vi "Process.vi"(11 "Actor":refnum<class "Alarm Handler Actor.lvclass">) -> ()   [LabVIEW 2015, in "Alarm Handler Actor.lvclass"]
uses:
  Alarm Handler Actor.lvclass
  Re-use Libraries/Utility/UI/System Button (without mouse hover).ctl
  Re-use Libraries/Minimal Actor Framework/Actors/Base Actor/Actor/Front Panel State.ctl
  Alarm Handler Actor.lvclass/Alarm Handler Actor.ctl
  Re-use Libraries/Utility/Utility.lvlib
  Re-use Libraries/Minimal Actor Framework/Actors/Base Actor/Actor/Actor.lvclass
  Re-use Libraries/Minimal Actor Framework/Messaging/Message/Message.lvclass
panel:
  out "Detail":string
  in  "Acknowledge":T1
  out "Number Of Errors":i32
  in  "Alarms":i32(listbox)=-1
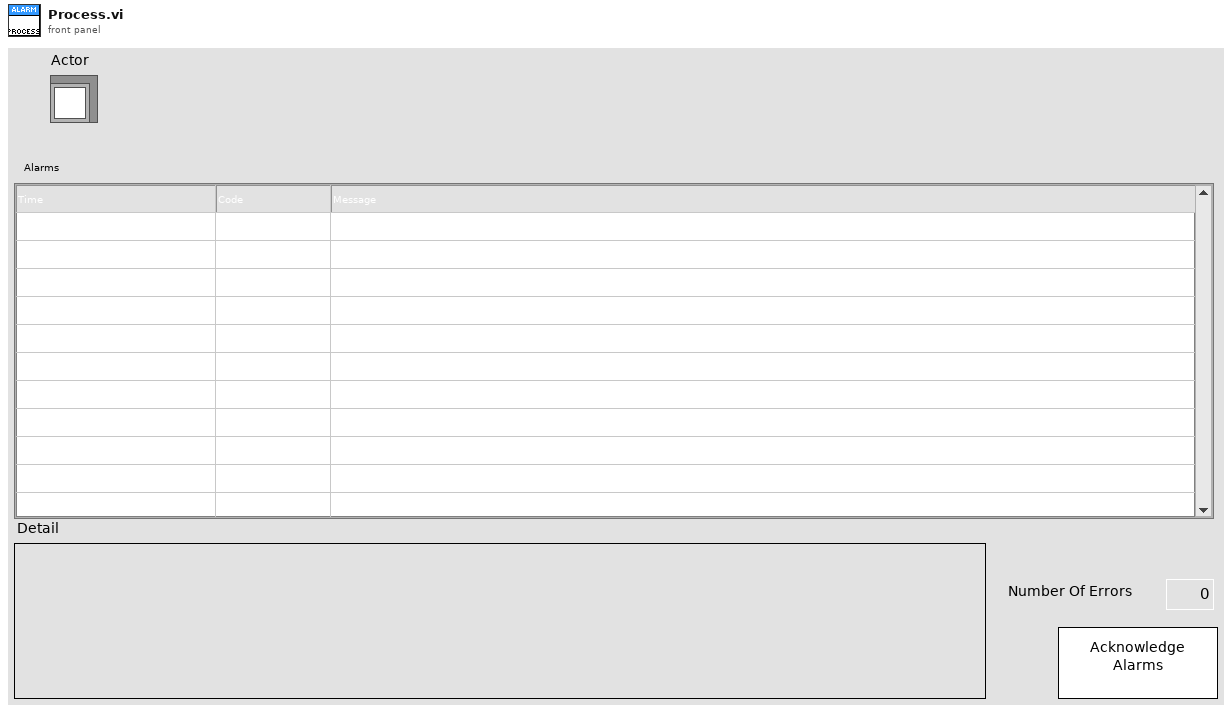
[diagram p1: front panel]
types:
  T1 = typedef "Utility.lvlib/System Button (without mouse hover).ctl" = bool
  T2 = typedef "Actor.lvclass/Front Panel State.ctl" = enum32{"Invalid", "Standard", "Closed", "Hidden", "Minimized", "Maximized"}
  T3 = typedef "LVPoint32TypeDef.ctl" = cluster{"Horizontal":i32, "Vertical":i32}
  T4 = typedef "LVRowAndColumnTypeDef.ctl" = cluster{"Row":i32, "Column":i32}
  T5 = typedef "Alarm Handler Actor.lvclass/Active Alarm.ctl" = cluster{"Alarm Detail":T6, "Count":i32, "First Error":timestamp, "Last Error":timestamp, "LabVIEW Error":bool}
  T6 = typedef "Alarm Handler Actor.lvclass/Alarm Details.ctl" = cluster{"Code":i32, "Loop":i32, "Description":string, "Severity":i32, "Clear on Ack?":bool, "Log All Events?":bool}
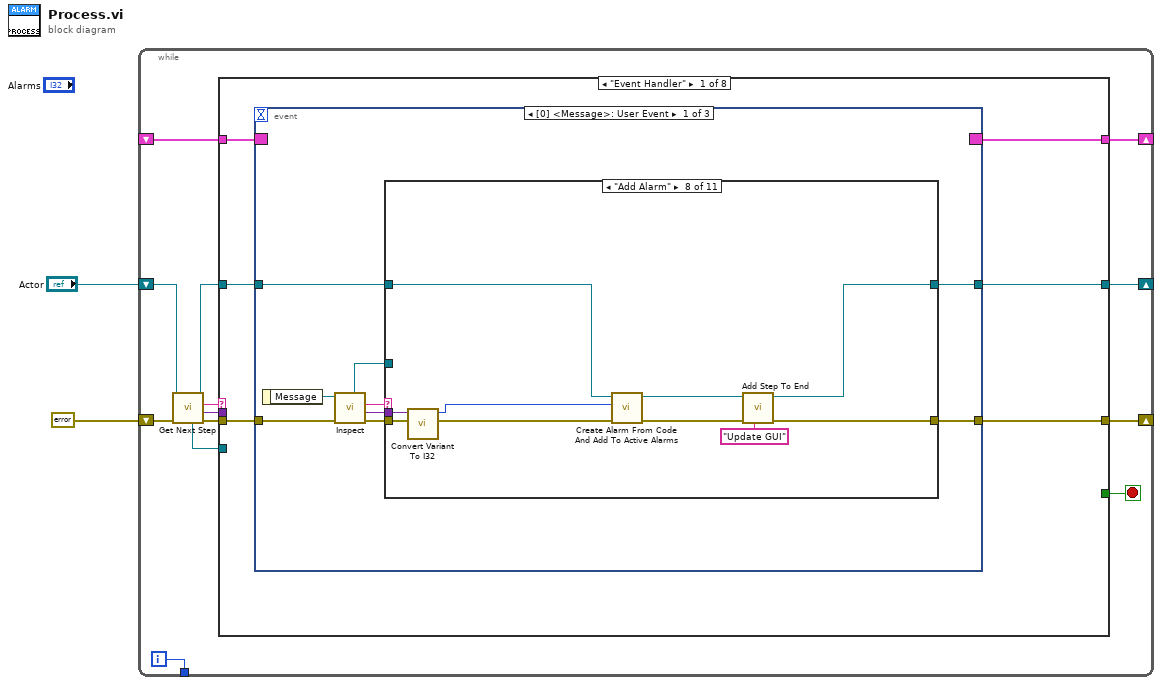
[diagram p0: block diagram]
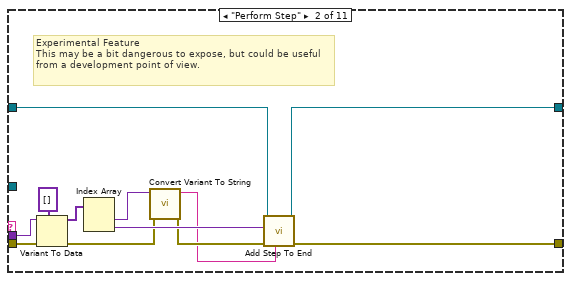
[diagram p3: hidden frame]
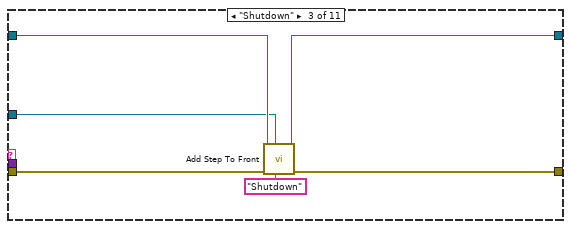
[diagram p4: hidden frame]
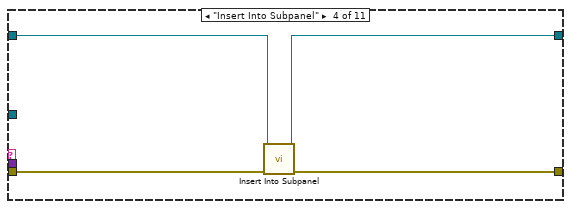
[diagram p5: hidden frame]
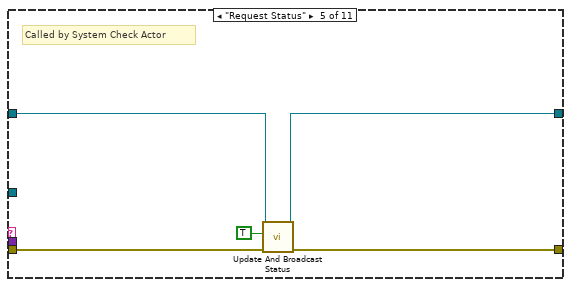
[diagram p6: hidden frame]
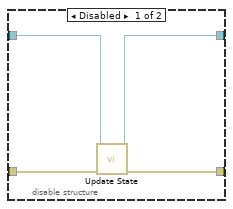
[diagram p8: hidden frame]
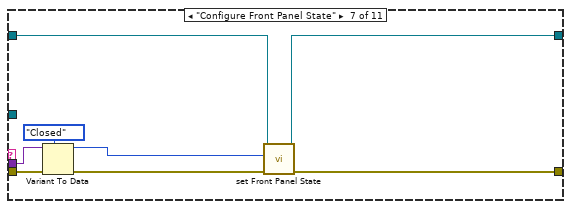
[diagram p9: hidden frame]
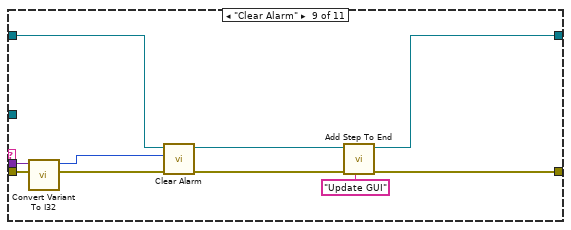
[diagram p10: hidden frame]
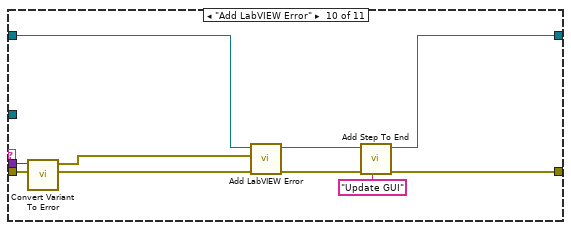
[diagram p11: hidden frame]
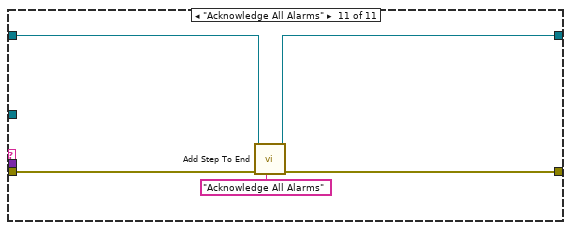
[diagram p12: hidden frame]
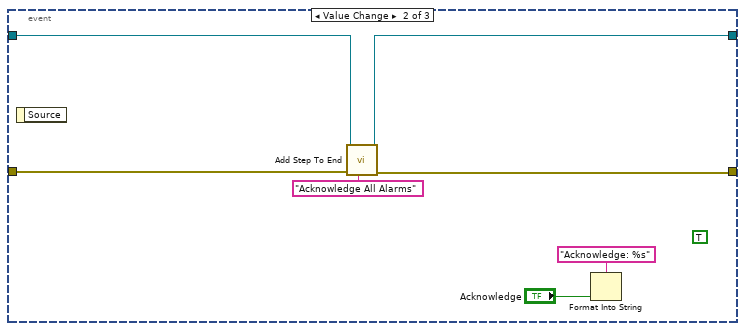
[diagram p13: hidden frame]
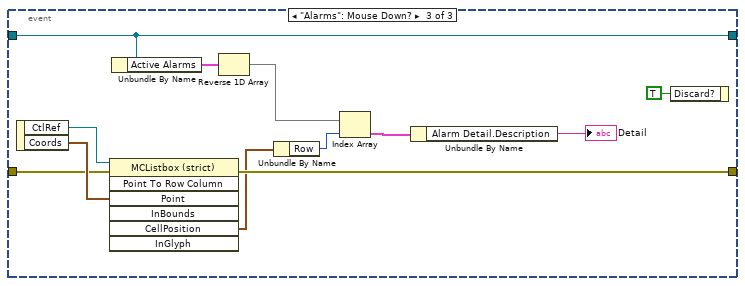
[diagram p14: hidden frame]
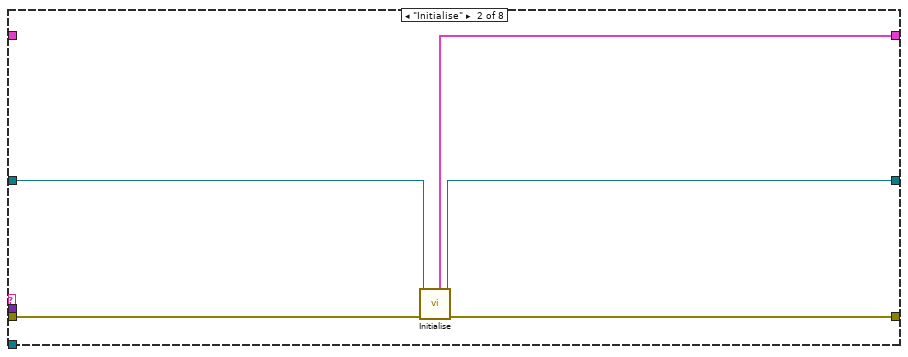
[diagram p15: hidden frame]
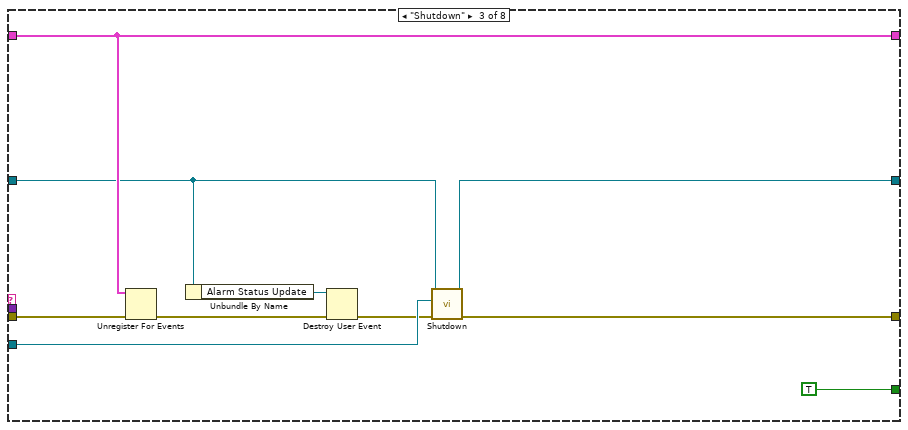
[diagram p16: hidden frame]
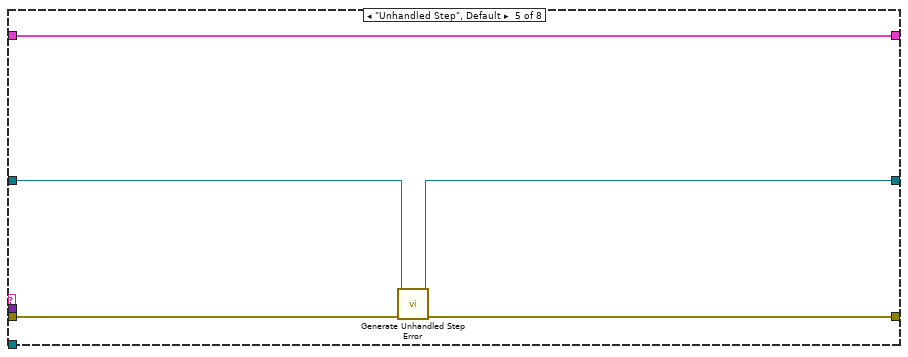
[diagram p18: hidden frame]
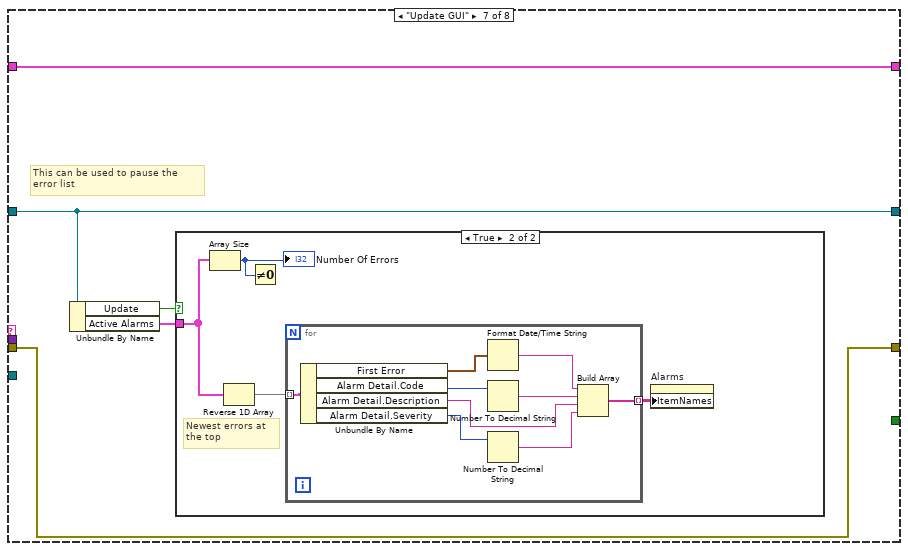
[diagram p20: hidden frame]
diagram:
  n1 = while {
    shift-right: [w4] -> _
    shift-left: "Actor" -> [w3]
    shift-right: [w11] -> _
    shift-left: _ -> [w10]
    shift-right: [w8] -> _
    shift-left: errorcluster {"status"=FALSE, "code"=0, "source"=""} ("error constant") -> [w7]
    tunnel: [w6] -> _
    i -> [w6]
    stop <- w15 stop-if-true
    n2 = call-dynamic "Get Next Step.vi"("error in (no error)"=w7, "Actor in"=w3) -> ("error out"=w9:errorcluster, "Parameter"=w12:variant, "Step"=w13:string, "Actor out"=w14:refnum<class "Alarm Handler Actor.lvclass">, "Reply Channel"=w5:refnum<notifier>)  [unwired: 5 in]
    n3 = case shown="\"Event Handler\"" w13 {
      tunnel: [_ _ TRUE _ _ _ _ _] -> w15
      tunnel: w14 -> [w21 w136 w139 w147 w153 w155 w159 w182]
      tunnel: [w16 w132 w141 w147 w150 w155 w159 w177] -> w4
      tunnel: w12 -> [_ _ _ _ _ _ _ _]
      tunnel: [w19 w133 w145 w149 w154 w157 w162 w185] -> w11
      tunnel: w10 -> [w20 _ w145 w149 w154 w157 w162 w185]
      tunnel: w9 -> [w18 w135 w144 w148 w152 w156 w158 w176]
      tunnel: [w17 w134 w142 w148 w151 w156 w158 w179] -> w8
      tunnel: w5 -> [_ _ w140 _ _ _ _ _]
      frame "Event Handler" {
        n4 = event shown="[0] <Message>: User Event" {
          selector: w20 -> [_ _ _]
          dyn-events: [_ _ _] -> w19
          timeout: _ -> [_ _ _]
          tunnel: w21 -> [w30 w116 w126]
          tunnel: [w29 w113 w126] -> w16
          tunnel: w18 -> [w27 w119 w127]
          tunnel: [w28 w115 w128] -> w17
          event User Event {
            n5 = event-data() -> ("Message"=w26:refnum<class "Message.lvclass">)  [unwired: 1 in]
            n6 = call "Inspect.vi"("error in (no error)"=w27, "Message in"=w26) -> ("error out"=w23:errorcluster, "Data"=w24:variant, "Name"=w25:string, "Reply Channel"=w22:refnum<notifier>)  [unwired: 5 in, 1 out]
            n7 = case shown="\"Add Alarm\"" w25 {
              tunnel: w30 -> [w32 w44 w50 w54 w58 w61 w77 w87 w91 w107 w112]
              tunnel: [w32 w43 w49 w53 w57 w60 w76 w79 w90 w98 w108] -> w29
              tunnel: w23 -> [w31 w41 w47 w52 w56 w63 w73 w86 w94 w106 w111]
              tunnel: [w31 w42 w46 w51 w55 w62 w75 w78 w89 w100 w109] -> w28
              tunnel: w24 -> [_ w33 _ _ _ _ w74 w85 w93 w105 _]
              tunnel: w22 -> [_ _ w45 _ _ _ _ _ _ _ _]
              frame Default {
              }
              frame "Perform Step" {
                # "Experimental Feature\nThis may be a bit dangerous to expose, but could be useful from a development point of view."
                n8 = Variant To Data(error in=w41, type=variant[] [], Variant=w33) -> (data=w39:variant[], error out=w36:errorcluster)
                n9 = Index Array(array=w39) -> (element #1=w37:variant, element #2=w38:variant)  [unwired: 2 in]
                n10 = call "Convert Variant To String.vi"("error in (no error)"=w36, "Variant"=w37) -> ("error out"=w35:errorcluster, "String"=w34:string)  [unwired: 8 in]
                n11 = call-dynamic "Add Step To End.vi"("Step Name"=w34, "error in (no error)"=w35, "Parameter"=w38, "Actor in"=w44) -> ("error out"=w42:errorcluster, "Actor out"=w43:refnum<class "Alarm Handler Actor.lvclass">)  [unwired: 6 in]
              }
              frame "Shutdown" {
                n12 = call-dynamic "Add Step To Front.vi"("Step Name"="Shutdown", "Reply Channel"=w45, "error in (no error)"=w47, "Actor in"=w50) -> ("error out"=w46:errorcluster, "Actor out"=w49:refnum<class "Alarm Handler Actor.lvclass">)  [unwired: 6 in]
              }
              frame "Insert Into Subpanel" {
                n13 = call-dynamic "Insert Into Subpanel.vi"("error in (no error)"=w52, "Actor in"=w54) -> ("error out"=w51:errorcluster, "Actor out"=w53:refnum<class "Alarm Handler Actor.lvclass">)  [unwired: 8 in]
              }
              frame "Request Status" {
                # "Called by System Check Actor"
                n14 = call-dynamic "Update And Broadcast Status.vi"("error in (no error)"=w56, "OK"=TRUE, "Actor in"=w58) -> ("error out"=w55:errorcluster, "Actor out"=w57:refnum<class "Alarm Handler Actor.lvclass">)  [unwired: 7 in]
              }
              frame "State Update Tick" {
                # "Called by the Metronome"
                n15 = disable-structure shown="Enabled" {
                  disable-tunnel: w63 -> [w67 w68]
                  disable-tunnel: [w66 w68] -> w62
                  disable-tunnel: w61 -> [w65 w69]
                  disable-tunnel: [w64 w69] -> w60
                  frame Disabled {
                    n16 = call "Update State.vi"("error in (no error)"=w67, "Alarm Handler Actor in"=w65) -> ("error out"=w66:errorcluster, "Alarm Handler Actor out"=w64:refnum<class "Alarm Handler Actor.lvclass">)  [unwired: 8 in]
                  }
                  frame Enabled {
                    # "Metronome is not used in Alarm Handler.\n\nNo action here. Look at the System Check actor"
                  }
                }
              }
              frame "Configure Front Panel State" {
                n17 = Variant To Data(error in=w73, type=Front_Panel_State."Closed" ("Front Panel State"), Variant=w74) -> (data=w70:T2, error out=w72:errorcluster)
                n18 = call-dynamic "set Front Panel State.vi"("error in (no error)"=w72, "Front Panel State"=w70, "Actor in"=w77) -> ("error out"=w75:errorcluster, "Actor out"=w76:refnum<class "Alarm Handler Actor.lvclass">)  [unwired: 7 in]
              }
              frame "Add Alarm" {
                n19 = call "Convert Variant To I32.vi"("error in (no error)"=w86, "Variant"=w85) -> ("error out"=w84:errorcluster, "Numeric"=w83:i32)  [unwired: 8 in]
                n20 = call "Create Alarm From Code And Add To Active Alarms.vi"("error in (no error)"=w84, "Numeric"=w83, "Alarm Handler Actor in"=w87) -> ("error out"=w81:errorcluster, "Alarm Handler Actor out"=w80:refnum<class "Alarm Handler Actor.lvclass">)  [unwired: 7 in]
                n21 = call-dynamic "Add Step To End.vi"("Step Name"="Update GUI", "error in (no error)"=w81, "Actor in"=w80) -> ("error out"=w78:errorcluster, "Actor out"=w79:refnum<class "Alarm Handler Actor.lvclass">)  [unwired: 7 in]
              }
              frame "Clear Alarm" {
                n22 = call "Convert Variant To I32.vi"("error in (no error)"=w94, "Variant"=w93) -> ("error out"=w92:errorcluster, "Numeric"=w88:i32)  [unwired: 8 in]
                n23 = call "Clear Alarm.vi"("error in (no error)"=w92, "Alarm Code"=w88, "Alarm Handler Actor in"=w91) -> ("error out"=w97:errorcluster, "Alarm Handler Actor out"=w95:refnum<class "Alarm Handler Actor.lvclass">)  [unwired: 7 in]
                n24 = call-dynamic "Add Step To End.vi"("Step Name"="Update GUI", "error in (no error)"=w97, "Actor in"=w95) -> ("error out"=w89:errorcluster, "Actor out"=w90:refnum<class "Alarm Handler Actor.lvclass">)  [unwired: 7 in]
              }
              frame "Add LabVIEW Error" {
                n25 = call "Convert Variant To Error.vi"("error in (no error)"=w106, "Variant"=w105) -> ("error out"=w103:errorcluster, "Error"=w104:errorcluster)  [unwired: 8 in]
                n26 = call "Add LabVIEW Error.vi"("error in (no error)"=w103, "LabVIEW Error"=w104, "Alarm Handler Actor in"=w107) -> ("error out"=w101:errorcluster, "Alarm Handler Actor out"=w99:refnum<class "Alarm Handler Actor.lvclass">)  [unwired: 7 in]
                n27 = call-dynamic "Add Step To End.vi"("Step Name"="Update GUI", "error in (no error)"=w101, "Actor in"=w99) -> ("error out"=w100:errorcluster, "Actor out"=w98:refnum<class "Alarm Handler Actor.lvclass">)  [unwired: 7 in]
              }
              frame "Acknowledge All Alarms" {
                n28 = call-dynamic "Add Step To End.vi"("Step Name"="Acknowledge All Alarms", "error in (no error)"=w111, "Actor in"=w112) -> ("error out"=w109:errorcluster, "Actor out"=w108:refnum<class "Alarm Handler Actor.lvclass">)  [unwired: 7 in]
              }
            }
          }
          event Value Change {
            (unwired) TRUE
            n29 = event-data() -> ()  [unwired: 1 in, 1 out]
            n30 = call-dynamic "Add Step To End.vi"("Step Name"="Acknowledge All Alarms", "error in (no error)"=w119, "Actor in"=w116) -> ("error out"=w115:errorcluster, "Actor out"=w113:refnum<class "Alarm Handler Actor.lvclass">)  [unwired: 7 in]
            n31 = Format Into String(format string="Acknowledge: %s", "Acknowledge") -> ()  [unwired: 2 in, 2 out]
          }
          event "Alarms": Mouse Down? {
            n32 = event-data() -> ("CtlRef"=w130:refnum<vi>, "Coords"=w129:T3)  [unwired: 1 in]
            n33 = invoke class="MCListbox (strict)" method="Point To Row Column"(reference=w130, error in=w127, "Point"=w129) -> (error out=w128:errorcluster, "CellPosition"=w125:T4)  [unwired: 4 in, 5 out]
            n34 = Unbundle By Name(w126) -> ("Active Alarms"=w121:T5[])
            n35 = Reverse 1D Array(array=w121) -> (reversed array=w120:T5[])
            n36 = Unbundle By Name(w125) -> ("Row"=w124:i32)
            n37 = Index Array(array=w120, index=w124) -> (element=w123:T5)
            n38 = Unbundle By Name(w123) -> ("Alarm Detail.Description"=→"Detail":string)
            n39 = event-data("Discard?"=TRUE) -> ()  [unwired: 1 in, 1 out]
          }
        }
      }
      frame "Initialise" {
        n40 = call "Initialise.vi"("error in (no error)"=w135, "Actor in"=w136) -> ("error out"=w134:errorcluster, "Actor out"=w132:refnum<class "Alarm Handler Actor.lvclass">, "Observers"=w133:cluster{"Actor":refnum<event-registration>})  [unwired: 7 in]
      }
      frame "Shutdown" {
        n41 = Unregister For Events(event registration refnum=w145, error in=w144) -> (error out=w138:errorcluster)
        n42 = Unbundle By Name(w139) -> ("Alarm Status Update"=w143:refnum<user-event>)
        n43 = Destroy User Event(user event=w143, error in=w138) -> (error out=w137:errorcluster)
        n44 = call-dynamic "Shutdown.vi"("error in (no error)"=w137, "Reply Channel"=w140, "Actor in"=w139) -> ("error out"=w142:errorcluster, "Actor out"=w141:refnum<class "Alarm Handler Actor.lvclass">)  [unwired: 7 in]
      }
      frame "Error Handler" {
        # "Don't really want the error handler to add more errors!\n\nHopefully this state will never occur."
      }
      frame "Unhandled Step", Default {
        n45 = call-dynamic "Generate Unhandled Step Error.vi"("error in (no error)"=w152, "Actor in"=w153) -> ("error out"=w151:errorcluster, "Actor out"=w150:refnum<class "Alarm Handler Actor.lvclass">)  [unwired: 8 in]
      }
      frame "-----------------------" {
        # "Separator"
      }
      frame "Update GUI" {
        # "This can be used to pause the error list"
        n46 = Unbundle By Name(w159) -> ("Update"=w160:bool, "Active Alarms"=w161:T5[])
        n47 = case shown="True" w160 {
          tunnel: w161 -> [_ w164]
          frame False {
          }
          frame True {
            # "Newest errors at the top"
            n48 = Array Size(array=w164) -> (size(s)=w163:i32)
            "Number Of Errors" <- w163
            n49 = Reverse 1D Array(array=w164) -> (reversed array=w165:T5[])
            n50 = Not Equal To 0?(x=w163) -> ()  [unwired: 1 out]
            n51 = for {
              tunnel: [w173] -> w166 mode=indexing
              tunnel: w165 -> [w171] mode=indexing
              n52 = Unbundle By Name(w171) -> ("First Error"=w167:timestamp, "Alarm Detail.Code"=w170:i32, "Alarm Detail.Description"=w169:string, "Alarm Detail.Severity"=w168:i32)
              n53 = Format Date/Time String(seconds (now)=w167) -> (date/time string=w175:string)  [unwired: 2 in]
              n54 = Number To Decimal String(number=w170) -> (decimal integer string=w174:string)  [unwired: 1 in]
              n55 = Number To Decimal String(number=w168) -> (decimal integer string=w172:string)  [unwired: 1 in]
              n56 = Build Array(w175, w174, w169, w172) -> (w173:string[])
            }
            n57 = property on="Alarms" class="MCListbox (strict)"("ItemNames"=w166) -> ()  [unwired: 2 in, 2 out]
          }
        }
      }
      frame "Acknowledge All Alarms" {
        n58 = call "Clear LabVIEW Errors.vi"("error in (no error)"=w176, "Alarm Handler Actor in"=w182) -> ("error out"=w184:errorcluster, "Alarm Handler Actor out"=w183:refnum<class "Alarm Handler Actor.lvclass">)  [unwired: 8 in]
        n59 = call "Clear GUI Errors.vi"("error in (no error)"=w184, "Alarm Handler Actor in"=w183) -> ("error out"=w180:errorcluster, "Alarm Handler Actor out"=w178:refnum<class "Alarm Handler Actor.lvclass">)  [unwired: 8 in]
        n60 = call-dynamic "Add Step To End.vi"("Step Name"="Update GUI", "error in (no error)"=w180, "Actor in"=w178) -> ("error out"=w179:errorcluster, "Actor out"=w177:refnum<class "Alarm Handler Actor.lvclass">)  [unwired: 7 in]
      }
    }
  }
